vi "Handle Error.vi"(8 "error in":errorcluster, 11 "SMO":refnum<class "SMO.lvclass">) -> (0 "handling error":errorcluster, 2 "Unhandled error":errorcluster, 3 "SMO out":refnum<class "SMO.lvclass">)   [LabVIEW 2013, in "SMO.lvclass"]
uses:
  SMO.lvclass
panel:
  # "For instructions on how to use the JKI State Machine Objects, examples and video tutorials, visit:\nhttp://jki.net/state-machine-objects/\n\nJKI State Machine Objects™\nhttp://jki.net/state-machine-objects/\nCopyright (C) 2005-2015, JKI <info@jki.net>\nALL RIGHTS RESERVED"
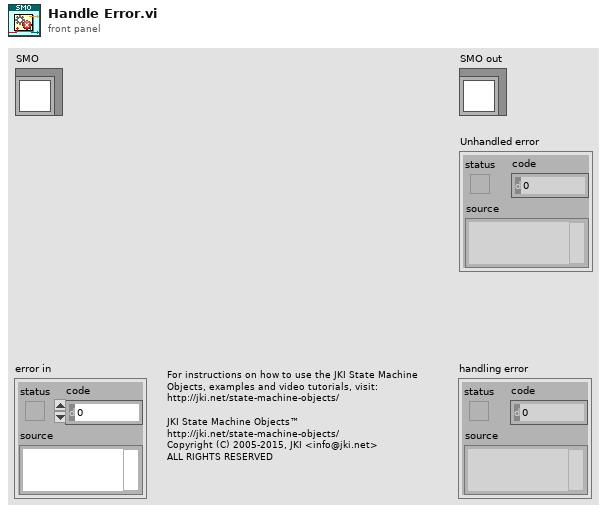
[diagram p1: front panel]
types:
  T1 = typedef "SMO.lvclass/Public Events.ctl" = cluster{"Error":refnum<user-event>}
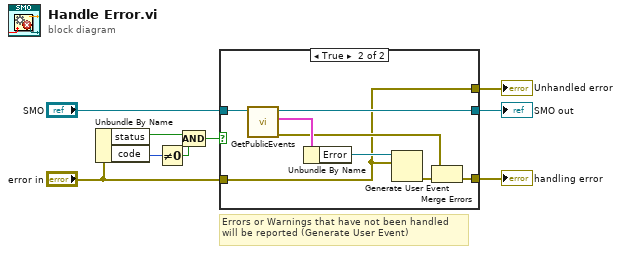
[diagram p0: block diagram]
diagram:
  # "Errors or Warnings that have not been handled\nwill be reported (Generate User Event)"
  n1 = Unbundle By Name("error in") -> ("status"=w7:bool, "code"=w6:i32)
  n2 = Not Equal To 0?(x=w6) -> (x != 0?=w4:bool)
  n3 = Compound Arithmetic op=AND(w7, w4) -> (w5:bool)
  n4 = case shown="True" w5 {
    tunnel: "SMO" -> [w11 w19]
    tunnel: [w11 w18] -> w9
    tunnel: [_ w15] -> w8
    tunnel: "error in" -> [w10 w12]
    tunnel: [w10 w12] -> w1
    frame False {
    }
    frame True {
      n5 = call "GetPublicEvents.vi"("SMO"=w19) -> ("error out"=w14:errorcluster, "Public Events"=w17:T1, "SMO out"=w18:refnum<class "SMO.lvclass">)  [unwired: 8 in]
      n6 = Unbundle By Name(w17) -> ("Error"=w16:refnum<user-event>)
      n7 = Generate User Event(user event=w16, event data cluster=w12) -> (error out=w13:errorcluster)  [unwired: 2 in, 1 out]
      n8 = Merge Errors(w14, w13) -> (w15:errorcluster)
    }
  }
  "handling error" <- w8
  "SMO out" <- w9
  "Unhandled error" <- w1
